vi "Init Links.vi"(4 "L4":dbl=0.1136 format="%#_13g", 6 "L3":dbl=0.135, 7 "L2":dbl=0.155, 8 "error in (no error)":errorcluster, 9 "L1z":dbl=0.11, 10 "L1x":dbl=0.033, 11 "NI_Robotics_5R Type 1 Serial Arm Class in":refnum<class "NI_Robotics_5R Type 1 Serial Arm Class.lvclass">) -> (0 "error out":errorcluster, 3 "NI_Robotics_5R Type 1 Serial Arm Class out":refnum<class "NI_Robotics_5R Type 1 Serial Arm Class.lvclass">)   [LabVIEW 2017, in "NI_Robotics_5R Type 1 Serial Arm Class.lvclass"]
uses:
  <vilib>/robotics/Kinematics/Analytical/5R/Type 1/NI_Robotics_5R Type 1 Serial Arm Class.lvclass
  c:/Program Files (x86)/National Instruments/LabVIEW 2017/vi.lib/robotics/Kinematics/Robot/NI_Robotics_Serial Robot Arm.lvclass
  <vilib>/robotics/Kinematics/Analytical/5R/Type 1/NI_Robotics_5R Type 1 Serial Arm Class.lvclass/NI_Robotics_5R Type 1 Serial Arm Class.ctl
  <vilib>/robotics/Kinematics/DH Kinematic Parameters.ctl
  <vilib>/robotics/Kinematics/Link/Joint Type.ctl
  <vilib>/robotics/Kinematics/Link/NI_Robotics_Link.lvclass
  <vilib>/robotics/Kinematics/Robot/NI_Robotics_Serial Robot Arm.lvclass
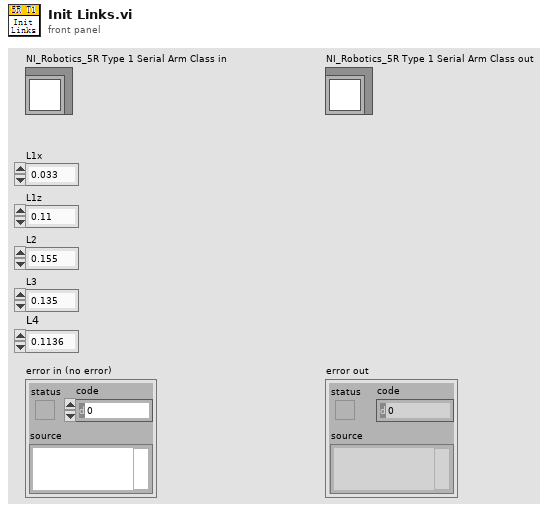
[diagram p1: front panel]
types:
  T1 = typedef "DH Kinematic Parameters.ctl" = cluster{"twist angle":dbl, "length":dbl, "rotation angle":dbl, "offset distance":dbl, "joint type":T2, "joint coordinate offset":dbl}
  T2 = typedef "NI_Robotics_Link.lvclass/Joint Type.ctl" = enum16{"Revolute", "Prismatic"}
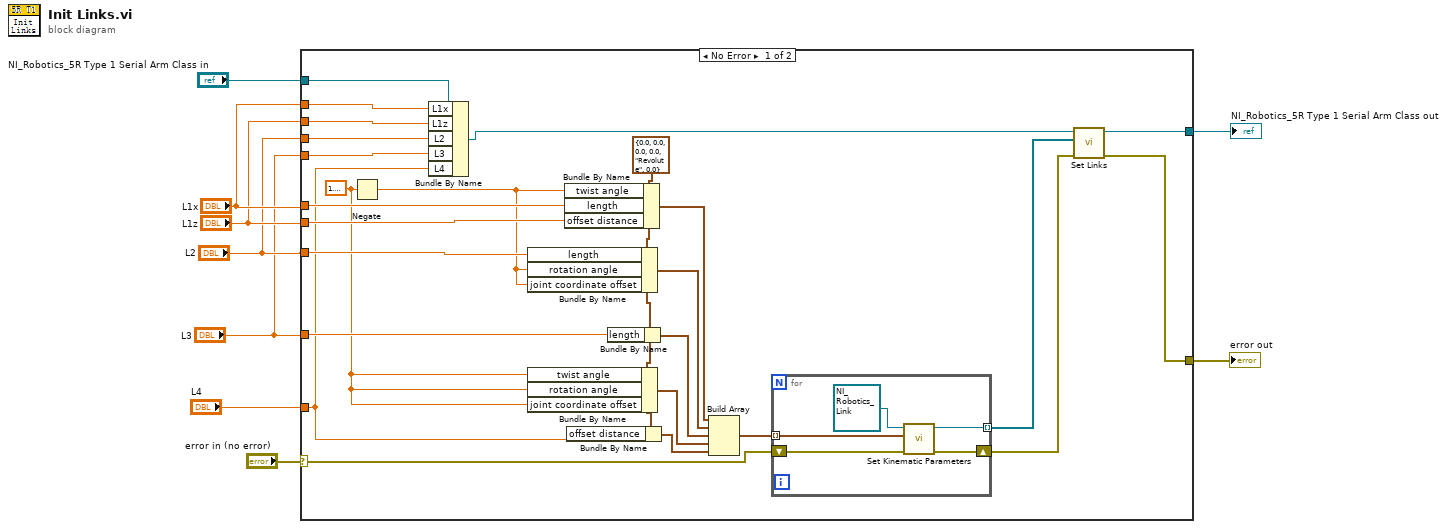
[diagram p0: block diagram]
diagram:
  n1 = case shown="No Error" "error in (no error)" {
    selector: "error in (no error)" -> [w23 w40]
    tunnel: "L1x" -> [w28 _]
    tunnel: "L1z" -> [w27 _]
    tunnel: "L2" -> [w26 _]
    tunnel: "L3" -> [w25 _]
    tunnel: "NI_Robotics_5R Type 1 Serial Arm Class in" -> [w22 w41]
    tunnel: "L1x" -> [w21 _]
    tunnel: "L1z" -> [w20 _]
    tunnel: "L2" -> [w19 _]
    tunnel: "L3" -> [w18 _]
    tunnel: [w14 w41] -> w3
    tunnel: [w13 w40] -> w2
    tunnel: "L4" -> [w10 _]
    frame No Error {
      w11 = 1.5707963267948966
      w34 = T1 {"twist angle"=0.0, "length"=0.0, "rotation angle"=0.0, "offset distance"=0.0, "joint type"=enum."Revolute", "joint coordinate offset"=0.0} ("Link Parameters")
      n2 = Negate(x=w11) -> (-x=w12:dbl)
      n3 = Bundle By Name(cluster=w22, "L1x"=w21, "L1z"=w20, "L2"=w19, "L3"=w18, "L4"=w10) -> (w17:refnum<class "NI_Robotics_5R Type 1 Serial Arm Class.lvclass">)
      n4 = Bundle By Name(cluster=w34, "length"=w26, "rotation angle"=w12, "joint coordinate offset"=w12) -> (w32:T1)
      n5 = Bundle By Name(cluster=w34, "twist angle"=w11, "rotation angle"=w11, "joint coordinate offset"=w11) -> (w30:T1)
      n6 = Bundle By Name(cluster=w34, "twist angle"=w12, "length"=w28, "offset distance"=w27) -> (w33:T1)
      n7 = Bundle By Name(cluster=w34, "offset distance"=w10) -> (w29:T1)
      n8 = Bundle By Name(cluster=w34, "length"=w25) -> (w31:T1)
      n9 = Build Array(w33, w32, w31, w30, w29) -> (w24:T1[])
      n10 = for {
        tunnel: w24 -> [w37] mode=indexing
        shift-right: [w35] -> w15
        shift-left: w23 -> [w38]
        tunnel: [w36] -> w16 mode=indexing
        n11 = call <vilib>:"Set Kinematic Parameters.vi"("error in (no error)"=w38, "kinematic parameters"=w37, "link in"=refnum<class "NI_Robotics_Link.lvclass"> refnum ("Link")) -> ("error out"=w35:errorcluster, "link out"=w36:refnum<class "NI_Robotics_Link.lvclass">)  [unwired: 7 in]
      }
      n12 = call <vilib>:"Set Links.vi"("error in (no error)"=w15, "links"=w16, "serial arm in"=w17) -> ("error out"=w13:errorcluster, "serial arm out"=w14:refnum<class "NI_Robotics_5R Type 1 Serial Arm Class.lvclass">)  [unwired: 7 out]
    }
    frame Error {
    }
  }
  "error out" <- w2
  "NI_Robotics_5R Type 1 Serial Arm Class out" <- w3
